vi "PH_AxisGUI_6P.constructor.vi"(0 "name":string, 2 "data in":string, 5 "error in(no error)":errorcluster) -> (14 "i ref out":refnum<vi>, 16 "data out":string, 19 "error out":errorcluster)   [LabVIEW 2014, in "PH_AxisGUI_6P.lvlib"]
doc: "This class is forseen to control up to two Sixpack Axes (classes: Trinamic_Axis and Trinamic_Controller).\n\nThis class is part of the PHELIX user layer.\n\nauthor: Stefan Götte, GSI\n\nLicense Agreement for this software:\n\nCopyright (C)\nGesellschaft für Schwerionenforschung, GSI\nPlanckstr. 1\n64291 Darmstadt\nGermany\n\nContact: D.Beck@gsi.de \n\nThis program is free software; you can redistribute it and/or modify it under the terms of the \nGNU General Public License as published by the Free Software Foundation; either version 2 of \nthe license, or (at your option) any later version.\n\nThis program is distributed in the hope that it will be useful, but WITHOUT ANY WARRANTY; \nwithout even the implied warranty of MERCHANTABILITY or FITNESS FOR A PARTICULAR PURPOSE. See the GNU General License for more details (http://www.gnu.org).\n\nGesellschaft für Schwerionenforschung, GSI\nPlanckstr. 1, 64291 Darmstadt, Germany\nFor all questions and ideas contact: M.Richter@gsi.de, H.Brand@gsi.de or D.Beck@gsi.de.\nLast update: 16-JUN-2004"
uses:
  PH_AxisGUI_6P.lvlib
  PH_Basics/PH_AxisGUI_BaseClass/PH_AxisGUI_BaseClass.lvlib
  CS_Core/CSSystem/CSSystemLib/CSSystemLib.lvlib
  CS_Core/CSObj/CSObj.lvlib
  PH_Basics/PH_Class/PH_Class.lvlib
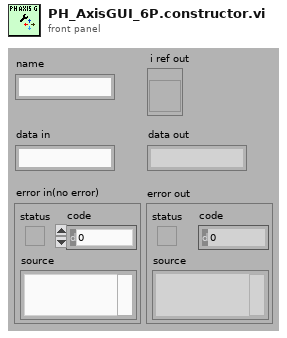
[diagram p1: front panel]
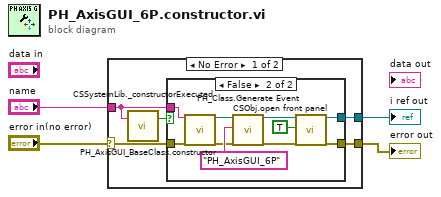
[diagram p0: block diagram]
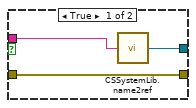
[diagram p2: hidden frame]
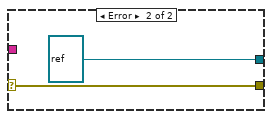
[diagram p3: hidden frame]
diagram:
  n1 = case shown="No Error" "error in(no error)" {
    selector: "error in(no error)" -> [w9 w24]
    tunnel: [w7 w24] -> w4
    tunnel: [w8 refnum<vi> refnum ("i ref out")] -> w3
    tunnel: "name" -> [w6 _]
    frame No Error {
      n2 = call "CSSystemLib._constructorExecuted.vi"("name"=w6) -> ("constructor executed?"=w5:bool)  [unwired: 18 in]
      n3 = case shown="False" w5 {
        tunnel: w9 -> [w10 w13]
        tunnel: [w11 w20] -> w8
        tunnel: [w10 w21] -> w7
        tunnel: w6 -> [w12 w22]
        frame True {
          n4 = call "CSSystemLib.name2ref.vi"("name"=w12) -> ("obj refnum"=w11:refnum<vi>)
        }
        frame False {
          n5 = call "PH_AxisGUI_BaseClass.constructor.vi"("name"=w22, "error in(no error)"=w13) -> ("i ref out"=w17:refnum<vi>, "error out"=w15:errorcluster)  [unwired: 15 in, 1 out]
          n6 = call "PH_Class.Generate Event.vi"("i ref in"=w17, "Class"="PH_AxisGUI_6P", "error in (no error)"=w15) -> ("i ref out"=w16:refnum<vi>, "error out"=w14:errorcluster)  [unwired: 15 in]
          n7 = call "CSObj.open front panel.vi"("i ref in"=w16, "frontPanelOpen"=TRUE ("front panel open"), "error in (no error)"=w14) -> ("i ref out"=w20:refnum<vi>, "error out"=w21:errorcluster)  [unwired: 15 in]
        }
      }
    }
    frame Error {
    }
  }
  "i ref out" <- w3
  "error out" <- w4
